vi "SignalGenerator.vi"(7 "error in (no error)":errorcluster, 8 "stop":bool, 9 "Amplitude":dbl, 10 "Frequency":dbl) -> (2 "error out":errorcluster)   [LabVIEW 2015]
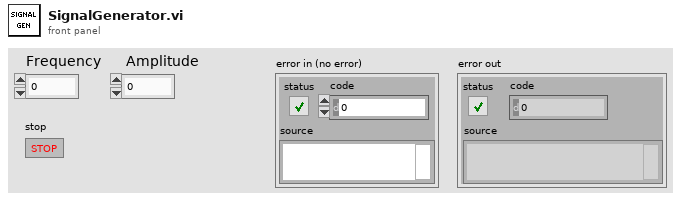
[diagram p1: front panel]
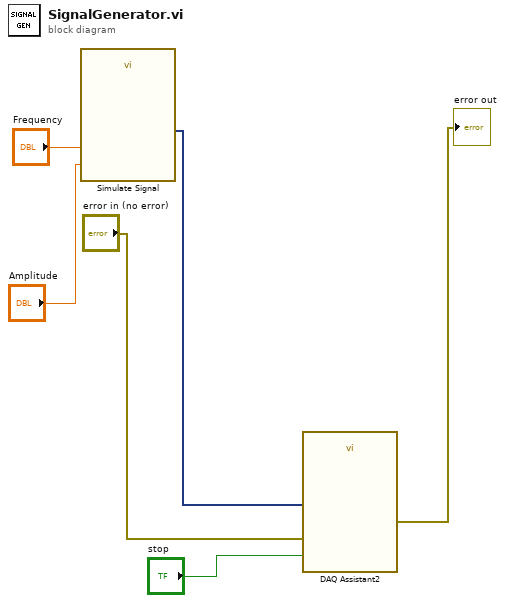
[diagram p0: block diagram]
diagram:
  n1 = call "Simulate Signal"("Frequency"="Frequency", "Amplitude"="Amplitude") -> ("Sine"=w4:dynamicdata)  [unwired: 12 in, 1 out]
  n2 = call "DAQ Assistant2"("data"=w4, "error in"="error in (no error)", "stop (F)"="stop") -> ("error out"=→"error out":errorcluster)  [unwired: 14 in, 2 out]
